vi "Filter2.vi"(8 "Number of points / scan":i32, 10 "Cut-off index":i16=50, 11 "Sigma":i16=5) -> (3 "Filter2":dbl[](array[numeric]))   [LabVIEW 2020]
uses:
  <vilib>/Analysis/2dsp.llb/Real FFT.vi
  <vilib>/Analysis/2dsp.llb/Inverse Real FFT.vi
  <vilib>/Analysis/NI_AALPro.lvlib
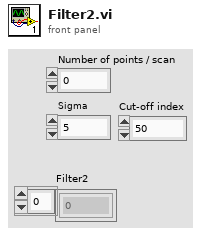
[diagram p1: front panel]
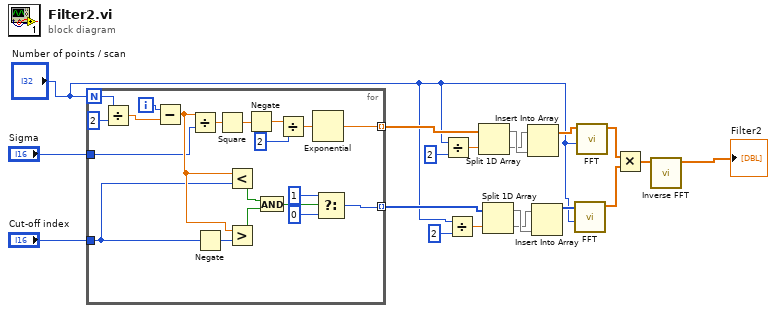
[diagram p0: block diagram]
diagram:
  n1 = for {
    N: "Number of points / scan" -> [w21]
    tunnel: [w29] -> w12 mode=indexing
    tunnel: [w28] -> w7 mode=indexing
    tunnel: "Sigma" -> [w23]
    tunnel: "Cut-off index" -> [w22]
    i -> [w20]
    n2 = Divide(x=w21, y=u8 2) -> (x/y=w33:dbl)
    n3 = Subtract(x=w20, y=w33) -> (x-y=w24:dbl)
    n4 = Divide(x=w24, y=w23) -> (x/y=w38:dbl)
    n5 = Negate(x=w22) -> (-x=w27:i16)
    n6 = Square(x=w38) -> (x^2=w37:dbl)
    n7 = Less?(x=w24, y=w22) -> (x < y?=w25:bool)
    n8 = Greater?(x=w24, y=w27) -> (0:w26:bool)
    n9 = Negate(x=w37) -> (-x=w36:dbl)
    n10 = And(x=w25, y=w26) -> (x .and. y?=w32:bool)
    n11 = Divide(x=w36, y=u8 2) -> (x/y=w34:dbl)
    n12 = Exponential(1:w34) -> (0:w29:dbl)
    n13 = Select(t=u8 1, s=w32, f=u8 0) -> (s? t:f=w28:u8)
  }
  n14 = Divide(x="Number of points / scan", y=u8 2) -> (x/y=w16:dbl)
  n15 = Divide(x="Number of points / scan", y=u8 2) -> (x/y=w11:dbl)
  n16 = Split 1D Array(array=w12, index=w16) -> (first subarray=w15:dbl[], second subarray=w14:dbl[])
  n17 = Split 1D Array(array=w7, index=w11) -> (first subarray=w10:u8[], second subarray=w9:u8[])
  n18 = Insert Into Array(array=w14, new element=w15) -> (w6:dbl[])  [unwired: 1 in]
  n19 = Insert Into Array(array=w9, new element=w10) -> (w5:u8[])  [unwired: 1 in]
  n20 = call-poly <vilib>:"FFT.vi"("FFT size"="Number of points / scan", "X"=w5) -> ("FFT {X}"=w18:cdb[])  [unwired: 8 in, 1 out]
  n21 = call-poly <vilib>:"FFT.vi"("FFT size"="Number of points / scan", "X"=w6) -> ("FFT {X}"=w19:cdb[])  [unwired: 8 in, 1 out]
  n22 = Multiply(x=w19, y=w18) -> (x*y=w17:cdb[])
  n23 = call-poly <vilib>:"Inverse FFT.vi"("FFT {X}"=w17) -> ("X"=→"Filter2":dbl[])  [unwired: 9 in, 1 out]
